vi "colouringTest.vi"() -> ()   [LabVIEW 2021]
uses:
  <vilib>/Utility/miscctls.llb/LVRGBAColorTypeDef.ctl
  <vilib>/picture/3D Picture Control/NI_3D Picture Control.lvlib
panel:
  in  "Material:Shininess":sgl min=0 max=128 step=16
  in  "specular":T1 {"Red" scale=0.0..1.0; "Green" scale=0.0..1.0; "Blue" scale=0.0..1.0; "Alpha" scale=0.0..1.0}
  in  "emission":T1 {"Red" scale=0.0..1.0; "Green" scale=0.0..1.0; "Blue" scale=0.0..1.0; "Alpha" scale=0.0..1.0}
  out "Array":string[](array[string])
  in  "Path":path
  out "3D Picture":refnum<vi>(3d-picture)
  in  "stop":bool
  in  "Selected object":i32
  out "Name":string
  out "Has Drawable?":bool
  in  "diffuse":T1 {"Red" scale=0.0..1.0; "Green" scale=0.0..1.0; "Blue" scale=0.0..1.0; "Alpha" scale=0.0..1.0}
  out "Objects totally":i32
  # "Colour seen outside lighting reflection cone"
  # "Colour shone out by object regardless of lighting"
  # "Colour emitted within reflection cone of lighting"
  # "High shininess limits the cone of specular reflections- makes a \"smoother mirror\""
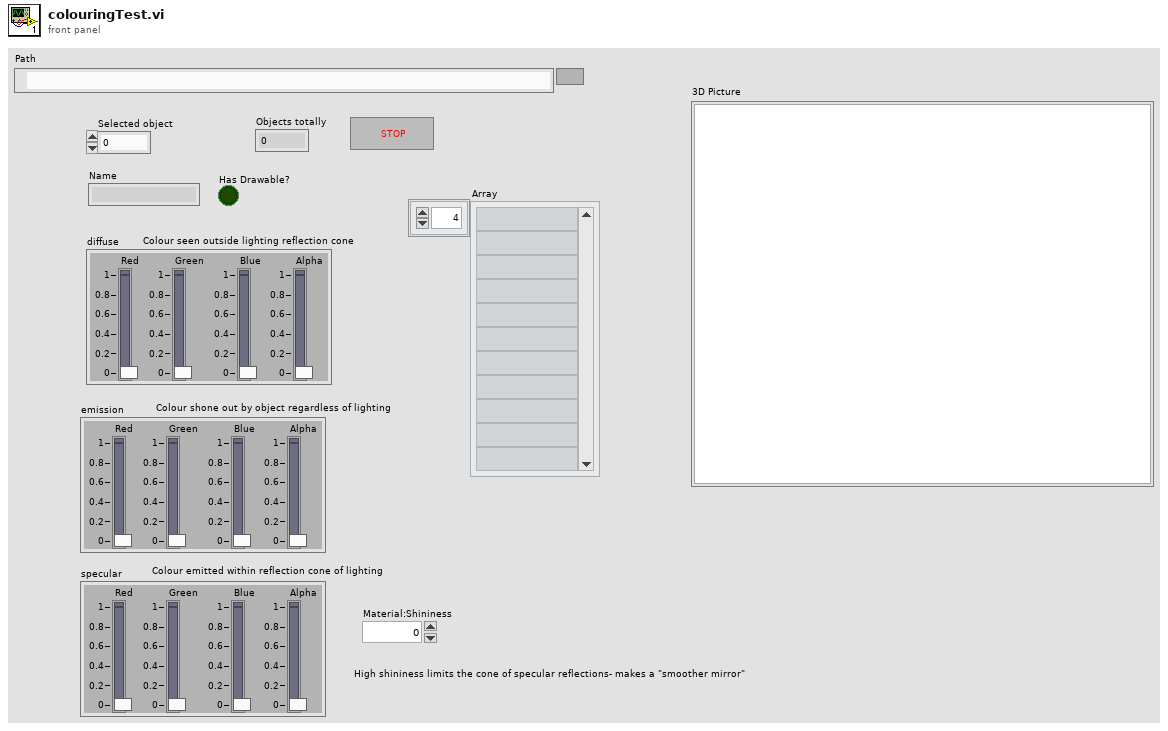
[diagram p1: front panel]
types:
  T1 = typedef "LVRGBAColorTypeDef.ctl" = cluster{"Red":sgl, "Green":sgl, "Blue":sgl, "Alpha":sgl}
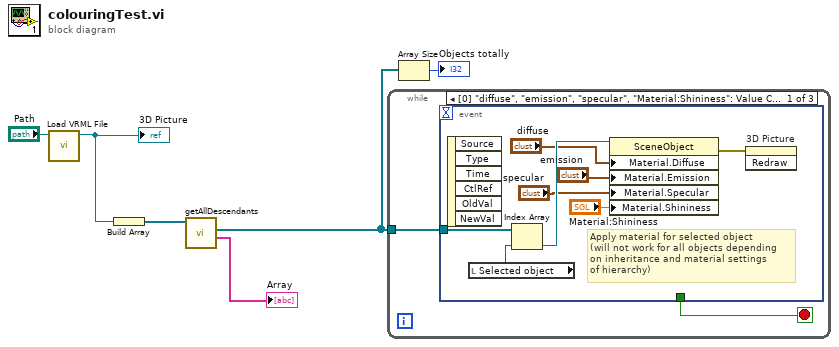
[diagram p0: block diagram]
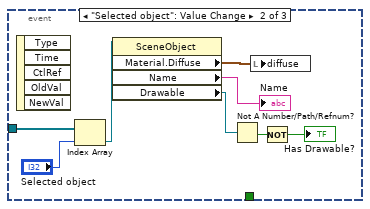
[diagram p2: hidden frame]
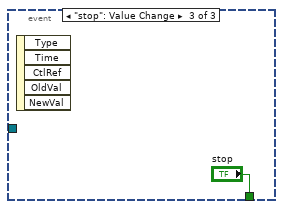
[diagram p3: hidden frame]
diagram:
  n1 = call <vilib>:"Load VRML File.vi"("Path"="Path") -> ("Scene:Read Scene File"=w3:refnum<vi>)  [unwired: 9 in, 1 out]
  "3D Picture" <- w3
  n2 = Build Array(w3) -> (w4:refnum<vi>[])
  n3 = call "getAllDescendants.vi"("parentsIn"=w4) -> ("allNames"=→"Array":string[], "allDescendants"=w5:refnum<vi>[])  [unwired: 9 in]
  n4 = while {
    tunnel: w5 -> [w8]
    stop <- w7 stop-if-true
    n5 = event shown="[0] \"diffuse\", \"emission\", \"specular\", \"Material:Shininess\": Value Change" {
      selector: _ -> [_ _ _]
      dyn-events: _ -> [_ _ _]
      timeout: _ -> [_ _ _]
      tunnel: w8 -> [w16 w24 _]
      tunnel: [_ _ "stop"] -> w7
      event "Material:Shininess": Value Change {
        # "Apply material for selected object\n(will not work for all objects depending\non inheritance and material settings\nof hierarchy)"
        n6 = event-data() -> ()  [unwired: 1 in, 6 out]
        n7 = local read "Selected object"() -> (w15:i32)
        n8 = Index Array(array=w16, index=w15) -> (element=w14:refnum<vi>)
        n9 = property class="SceneObject"(reference=w14, "Material.Diffuse"="diffuse", "Material.Emission"="emission", "Material.Specular"="specular", "Material.Shininess"="Material:Shininess") -> (error out=w13:errorcluster)  [unwired: 1 in, 1 out]
        n10 = invoke on="3D Picture" class="SceneGraphDisp (strict)" method="Redraw"(error in=w13) -> ()  [unwired: 2 in, 3 out]
      }
      event "Selected object": Value Change {
        n11 = event-data() -> ()  [unwired: 1 in, 5 out]
        n12 = Index Array(array=w24, index="Selected object") -> (element=w22:refnum<vi>)
        n13 = property class="SceneObject"(reference=w22) -> ("Material.Diffuse"=w21:T1, "Name"=→"Name":string, "Drawable"=w19:refnum<vi>)  [unwired: 1 in, 2 out]
        n14 = Not A Number/Path/Refnum?(number/path/refnum=w19) -> (NaN/Path/Refnum?=w18:bool)
        n15 = local write "diffuse"(w21) -> ()
        n16 = Not(x=w18) -> (.not. x?=→"Has Drawable?":bool)
      }
      event "stop": Value Change {
        n17 = event-data() -> ()  [unwired: 1 in, 5 out]
      }
    }
  }
  n18 = Array Size(array=w5) -> (size(s)=→"Objects totally":i32)
